vi "ImgSharpnessMetrics.vi"(9 "Image":T1, 10 "msk threshold":dbl=0.75 format="%#_13g", 11 "X":dbl[][](array[numeric])) -> (1 "Fourier space Display":T1(plugin-control), 3 "x/y":cdb)   [LabVIEW 2016]
uses:
  <vilib>/vision/Image Controls.llb/IMAQ Image.ctl
  <vilib>/Analysis/2dsp.llb/2D Real FFT.vi
  <vilib>/Analysis/NI_AALPro.lvlib
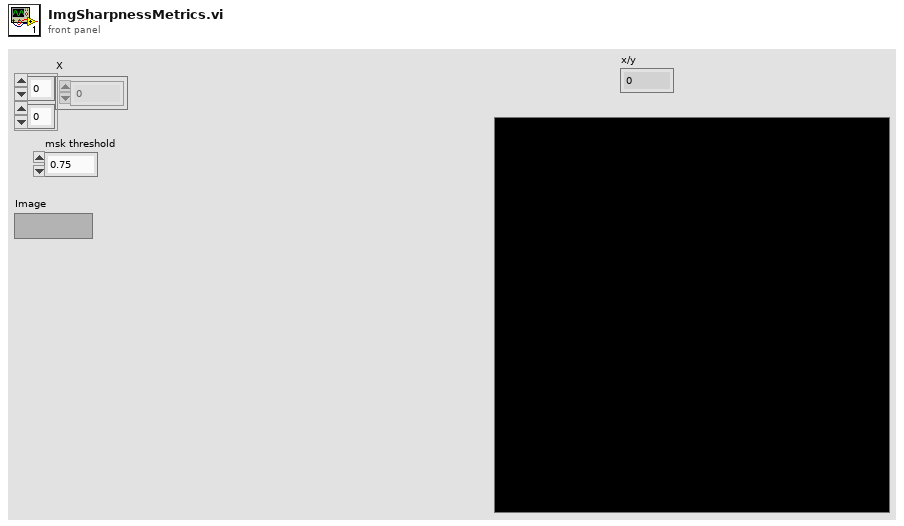
[diagram p1: front panel]
types:
  T1 = typedef "IMAQ Image.ctl" = refnum<image>
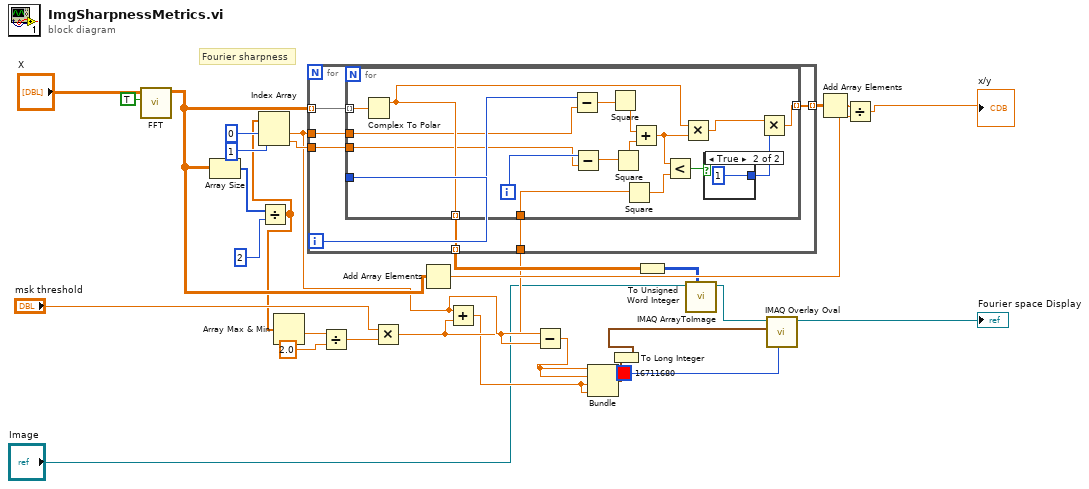
[diagram p0: block diagram]
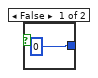
[diagram p2: hidden frame]
diagram:
  # "Fourier sharpness"
  n1 = call-poly <vilib>:"FFT.vi"("shift?"=TRUE, "X"="X") -> ("FFT {X}"=w24:cdb[][])  [unwired: 8 in, 1 out]
  n2 = Array Size(array=w24) -> (size(s)=w14:i32[])
  n3 = Divide(x=w14, y=2) -> (x/y=w13:dbl[])
  n4 = Index Array(array=w13, index #1=0 ("index"), index #2=1 ("index")) -> (element #1=w11:dbl, element #2=w12:dbl)
  n5 = Array Max & Min(array=w13) -> (min value=w18:dbl)  [unwired: 3 out]
  n6 = Divide(x=w18, y=2.0) -> (x/y=w20:dbl)
  n7 = Multiply(x="msk threshold", y=w20) -> (x*y=w10:dbl)
  n8 = for {
    tunnel: w24 -> [w36] mode=indexing
    tunnel: [w34] -> w27 mode=indexing
    tunnel: [w33] -> w23 mode=indexing
    tunnel: w11 -> [w32]
    tunnel: w12 -> [w31]
    tunnel: w10 -> [w30]
    i -> [w35]
    n9 = for {
      tunnel: w36 -> [w42] mode=indexing
      tunnel: w35 -> [w51]
      tunnel: [w44] -> w34 mode=indexing
      tunnel: [w41] -> w33 mode=indexing
      tunnel: w32 -> [w40]
      tunnel: w31 -> [w39]
      tunnel: w30 -> [w37]
      i -> [w53]
      n10 = Complex To Polar(r * e^(i*theta)=w42) -> (r=w41:dbl)  [unwired: 1 out]
      n11 = Subtract(x=w51, y=w40) -> (x-y=w50:dbl)
      n12 = Subtract(x=w53, y=w39) -> (x-y=w52:dbl)
      n13 = Square(x=w50) -> (x^2=w49:dbl)
      n14 = Square(x=w52) -> (x^2=w48:dbl)
      n15 = Square(x=w37) -> (x^2=w38:dbl)
      n16 = Add(x=w49, y=w48) -> (x+y=w43:dbl)
      n17 = Less?(x=w43, y=w38) -> (x < y?=w45:bool)
      n18 = Multiply(x=w41, y=w43) -> (x*y=w47:dbl)
      n19 = case shown="True" w45 {
        tunnel: [0 1] -> w46
        frame False {
        }
        frame True {
        }
      }
      n20 = Multiply(x=w47, y=w46) -> (x*y=w44:dbl)
    }
  }
  n21 = Add Array Elements(numeric array=w24) -> (sum=w29:cdb)
  n22 = Add(x=w11, y=w10) -> (x+y=w8:dbl)
  n23 = Subtract(x=w11, y=w10) -> (x-y=w9:dbl)
  n24 = Bundle(w9, w9, w8, w8) -> (w7:cluster{dbl, dbl, dbl, dbl})  [unwired: 1 in]
  n25 = To Long Integer(number=w7) -> (32bit integer=w6:cluster{i32, i32, i32, i32})
  n26 = To Unsigned Word Integer(number=w23) -> (unsigned 16bit integer=w22:u16[][])
  n27 = call "IMAQ ArrayToImage"("Image Pixels (U16)"=w22, "Image"="Image") -> ("Image Out"=w4:T1)  [unwired: 8 in, 1 out]
  n28 = call "IMAQ Overlay Oval"("Color"=u32 16711680, "Bounding Rectangle"=w6, "Image"=w4) -> ("Image Out"=→"Fourier space Display":T1)  [unwired: 7 in, 1 out]
  n29 = Add Array Elements(numeric array=w27) -> (sum=w26:dbl)
  n30 = Divide(x=w26, y=w29) -> (x/y=→"x/y":cdb)
